vi "Simulate PrtScr Key Press.vi"(8 "error in (no error)":errorcluster) -> (0 "error out":errorcluster)   [LabVIEW 2017, in "Error Dialog w Copy to Clipboard.lvlib"]
uses:
  Error Dialog w Copy to Clipboard.lvlib
  user32.dll
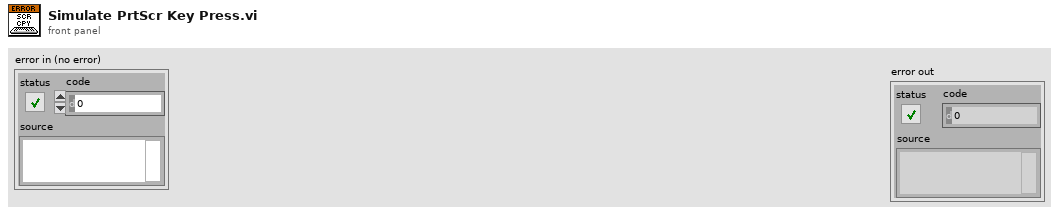
[diagram p1: front panel]
types:
  T1 = enum16{"Left Mouse Button", "Right Mouse Button", "Ctrl-Break", "Middle Mouse Button (3-button mice only)", "X1 mouse button (Win2k Only)", "X2 Mouse Button (Win2k Only)", "Undefined (1)", "BACKSPACE", "TAB", "Reserved (1)", "Reserved (2)", "CLEAR", "ENTER", "Undefined (2)", "Undefined (3)", "SHIFT", "CTRL", "ALT", "PAUSE", "CAPS LOCK", "IME Kana mode", "Undefined (4)", "IME Junja mode", "IME final mode", "IME Hanja mode", "IME Kanji mode", "Undefined    ", "ESC", "IME convert", "IME nonconvert", "IME accept", "IME mode change request", "SPACEBAR", "PAGE UP", "PAGE DOWN", "END", "HOME", "LEFT ARROW", "UP ARROW", "RIGHT ARROW", "DOWN ARROW", "SELECT", "PRINT", "EXECUTE", "PRINT SCREEN", "INS", "DEL", "HELP"}
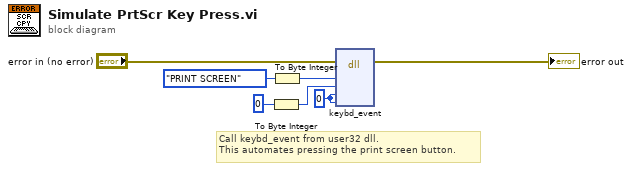
[diagram p0: block diagram]
diagram:
  w7 = 0 ("Input Value")
  # "Call keybd_event from user32 dll. \nThis automates pressing the print screen button."
  n1 = To Byte Integer(number=i16 0) -> (8bit integer=w5:i8)
  n2 = To Byte Integer(number=T1."PRINT SCREEN" ("Keyboard Stroke")) -> (8bit integer=w3:i8)
  n3 = dll-call lib="user32.dll" fn="keybd_event"(error in="error in (no error)", w3, w5, w7, w7) -> (error out=→"error out":errorcluster)  [unwired: 7 in, 1 out]
